vi "Delete Item in Tree.vi"(7 "Tree ref":refnum<vi>, 9 "Tree Move Indices":T1[](array[typedef]), 11 "TreeItems (current)":T2[](array[typedef])) -> (0 "error out":errorcluster)   [LabVIEW 2020, in "BetterDragAndDrop.lvlib" / "BetterTreeHandle.lvclass"]
uses:
  BetterTreeHandle/BetterTreeHandle.lvclass
  TreeItem.ctl
  Tree Move Indices.ctl
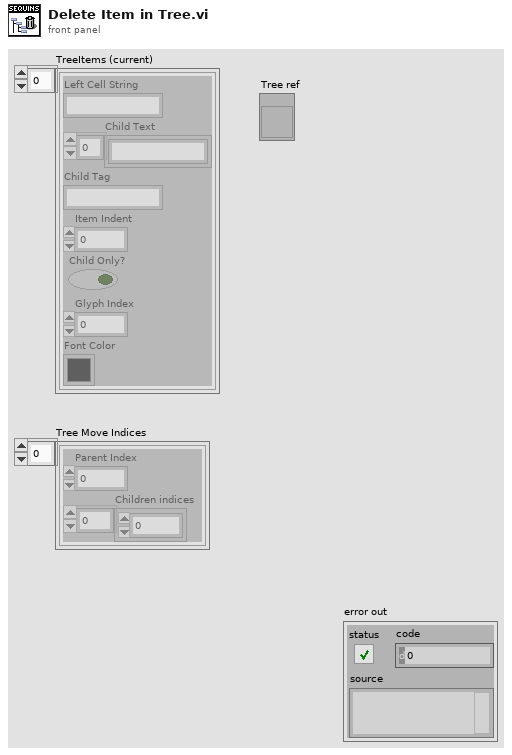
[diagram p1: front panel]
types:
  T1 = typedef "BetterDragAndDrop.lvlib/BetterTreeHandle.lvclass/Tree Move Indices.ctl" = cluster{"Parent Index":i32, "Children indices":i32[]}
  T2 = typedef "BetterDragAndDrop.lvlib/BetterTreeHandle.lvclass/TreeItem.ctl" = cluster{"Left Cell String":string, "Child Text":string[], "Child Tag":string, "Item Indent":i32, "Child Only?":bool, "Glyph Index":i32, "Font Color":u32}
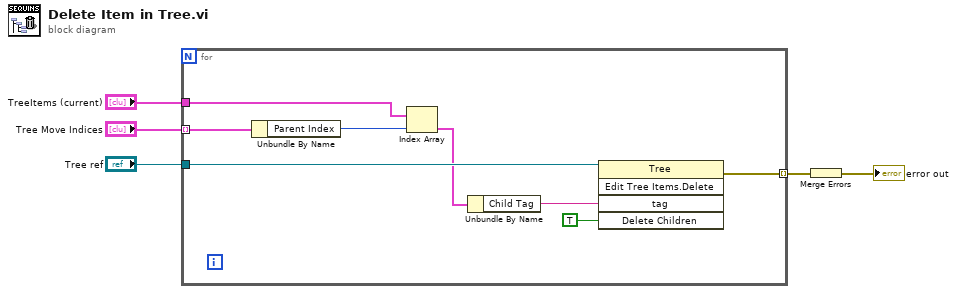
[diagram p0: block diagram]
diagram:
  n1 = for {
    tunnel: "Tree ref" -> [w13]
    tunnel: "Tree Move Indices" -> [w12] mode=indexing
    tunnel: "TreeItems (current)" -> [w9]
    tunnel: [w6] -> w2 mode=indexing
    n2 = Unbundle By Name(w12) -> ("Parent Index"=w8:i32)
    n3 = Index Array(array=w9, index=w8) -> (element=w11:T2)
    n4 = Unbundle By Name(w11) -> ("Child Tag"=w10:string)
    n5 = invoke class="Tree" method="Edit Tree Items.Delete"(reference=w13, "tag"=w10, "Delete Children"=TRUE ("Carry Children?")) -> (error out=w6:errorcluster)  [unwired: 2 in, 4 out]
  }
  n6 = Merge Errors(w2) -> (→"error out":errorcluster)
